vi "函数公式.vi"(6 "参数 b":dbl, 7 "参数 a":dbl, 8 "设定值 2":dbl, 9 "设定值 1":dbl) -> (0 "y2":dbl, 3 "y":dbl)   [LabVIEW 2010]
panel:
  in  "参数 c":dbl
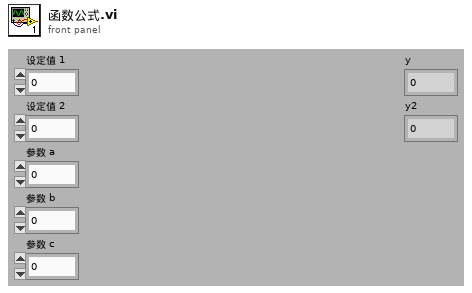
[diagram p1: front panel]
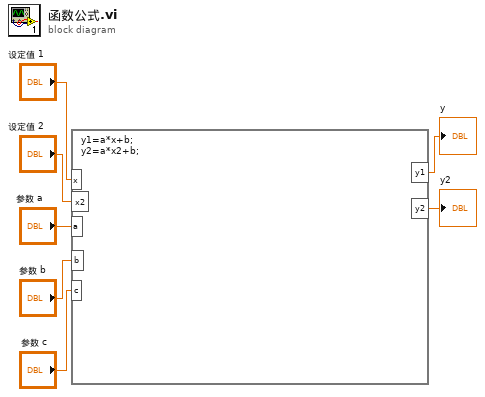
[diagram p0: block diagram]
diagram:
  n1 = formula code="y1=a*x+b;\ny2=a*x2+b;"("x"="设定值 1", "a"="参数 a", "b"="参数 b", "c"="参数 c", "x2"="设定值 2") -> ("y1"=→"y":dbl, "y2"=→"y2":dbl)
